vi "Draw Bone_picture.vi"(7 "Joints":refnum<k24>, 8 "error in":errorcluster, 9 "Ending Joint":i32(ring)=2 items=["SpineBase", "SpineMid", "Neck", "Head", "ShoulderLeft", "ElbowLeft", "WristLeft", "HandLeft", "ShoulderRight", "ElbowRight", "WristRight", "HandRight", "HipLeft", "KneeLeft", "AnkleLeft", "FootLeft", "HipRight", "KneeRight", "AnkleRight", "FootRight", "SpineShoulder", "HandTipLeft", "ThumbLeft", "HandTipRight", "ThumbRight"], 10 "Starting Joint":i32(ring)=3 items=["SpineBase", "SpineMid", "Neck", "Head", "ShoulderLeft", "ElbowLeft", "WristLeft", "HandLeft", "ShoulderRight", "ElbowRight", "WristRight", "HandRight", "HipLeft", "KneeLeft", "AnkleLeft", "FootLeft", "HipRight", "KneeRight", "AnkleRight", "FootRight", "SpineShoulder", "HandTipLeft", "ThumbLeft", "HandTipRight", "ThumbRight"], 11 "picture":picture) -> (0 "error out":errorcluster, 3 "picture out":picture)   [LabVIEW 2014]
uses:
  Microsoft.Kinect
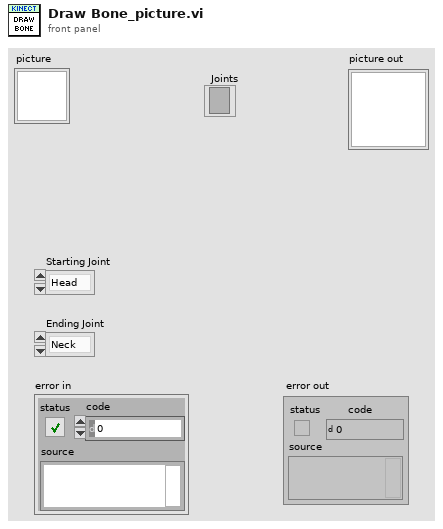
[diagram p1: front panel]
types:
  T1 = cluster{"Width":u16, "Style":enum32{"Solid", "Dash", "Dot", "DashDot", "DashDotDot"}}
  T2 = enum16{"Get Attribute", "Initialize", "Set Attribute"}
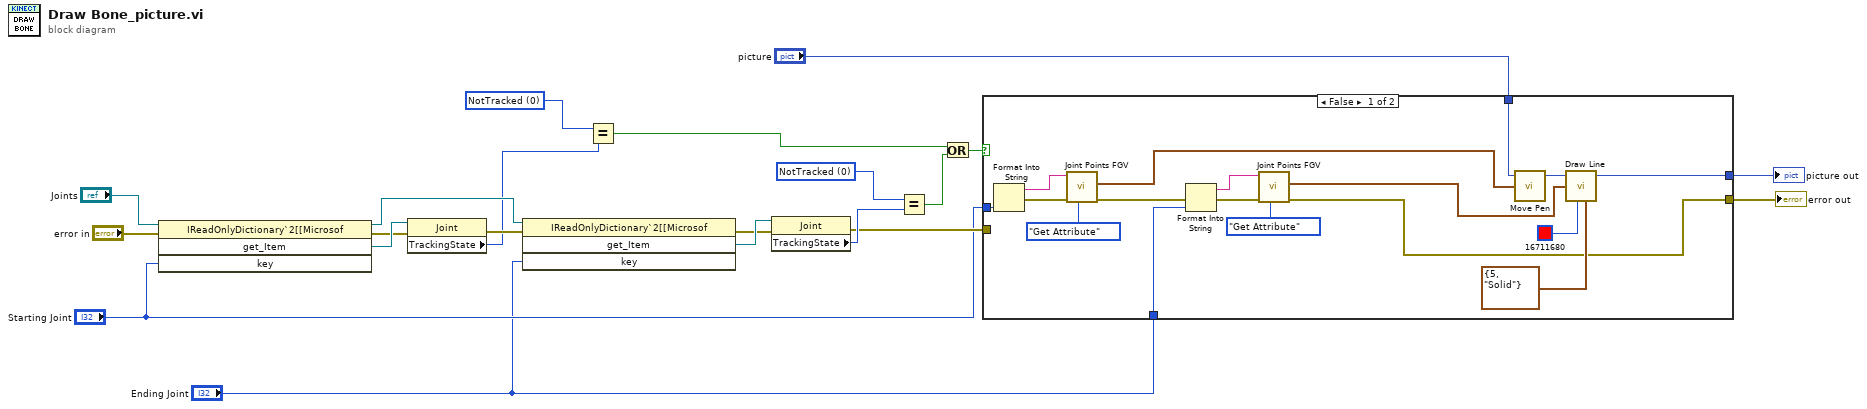
[diagram p0: block diagram]
diagram:
  w11 = 0 items=["NotTracked", "Inferred", "Tracked"] ("TrackingState")
  w13 = 0 items=["NotTracked", "Inferred", "Tracked"] ("TrackingState")
  n1 = invoke class="IReadOnlyDictionary`2[[Microsof" method="get_Item"(reference="Joints", error in="error in", "key"="Starting Joint") -> (reference out=w14:refnum<k24>, error out=w18:errorcluster, "get_Item"=w19:refnum<k24>)  [unwired: 1 in, 1 out]
  n2 = property class="Joint"(reference=w19, error in=w18) -> (error out=w15:errorcluster, "TrackingState"=w12:i32)  [unwired: 1 out]
  n3 = invoke class="IReadOnlyDictionary`2[[Microsof" method="get_Item"(reference=w14, error in=w15, "key"="Ending Joint") -> (error out=w16:errorcluster, "get_Item"=w17:refnum<k24>)  [unwired: 1 in, 2 out]
  n4 = Equal?(x=w13, y=w12) -> (x = y?=w7:bool)
  n5 = property class="Joint"(reference=w17, error in=w16) -> (error out=w6:errorcluster, "TrackingState"=w10:i32)  [unwired: 1 out]
  n6 = Equal?(x=w11, y=w10) -> (x = y?=w8:bool)
  n7 = Or(x=w7, y=w8) -> (x .or. y?=w9:bool)
  n8 = case shown="False" w9 {
    tunnel: "Starting Joint" -> [w37 _]
    tunnel: "Ending Joint" -> [w33 _]
    tunnel: [w24 w40] -> w21
    tunnel: w6 -> [_ w40]
    tunnel: "picture" -> [w23 w39]
    tunnel: [w22 w39] -> w1
    frame False {
      n9 = Format Into String(w37) -> (resulting string=w36:string, error out=w35:errorcluster)  [unwired: 3 in]
      n10 = call "Joint Points FGV.vi"("Command"=T2."Get Attribute", "error in (no error)"=w35, "name"=w36) -> ("error out"=w32:errorcluster, "Joint Point"=w28:cluster{"X":sgl, "Y":sgl})  [unwired: 7 in]
      n11 = Format Into String(error in=w32, w33) -> (resulting string=w31:string, error out=w34:errorcluster)  [unwired: 2 in]
      n12 = call "Joint Points FGV.vi"("Command"=T2."Get Attribute", "error in (no error)"=w34, "name"=w31) -> ("error out"=w24:errorcluster, "Joint Point"=w27:cluster{"X":sgl, "Y":sgl})  [unwired: 7 in]
      n13 = call <vilib>:"Move Pen.vi"("new position"=w28, "picture"=w23) -> ("new picture"=w29:picture)  [unwired: 3 in]
      n14 = call <vilib>:"Draw Line.vi"("picture"=w29, "end point"=w27, "color(black)"=u32 16711680, "pen"=T1 {"Width"=5, "Style"=enum."Solid"}) -> ("new picture"=w22:picture)  [unwired: 5 in]
    }
    frame True {
    }
  }
  "error out" <- w21
  "picture out" <- w1
